vi "y1y2 (子VI)-2.vi"(11 "Image Pixels (U8)输入":u8[][](array[numeric])) -> (0 "输出数组 2":cluster{i32, i32}[](array[cluster]), 2 "输出数组":cluster{i32, i32}[](array[cluster]))   [LabVIEW 2014]
panel:
  out "元素索引 2":i32
  out "元素索引":i32
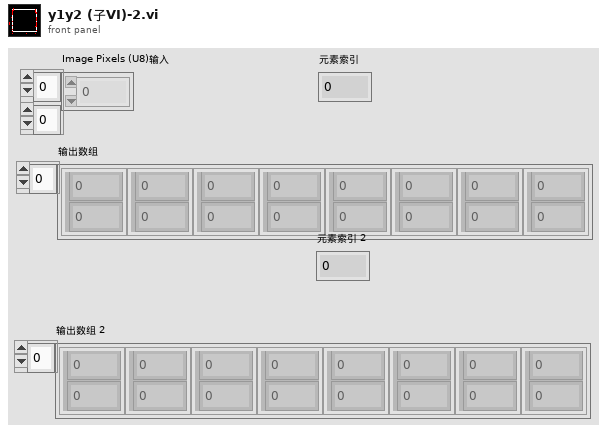
[diagram p1: front panel]
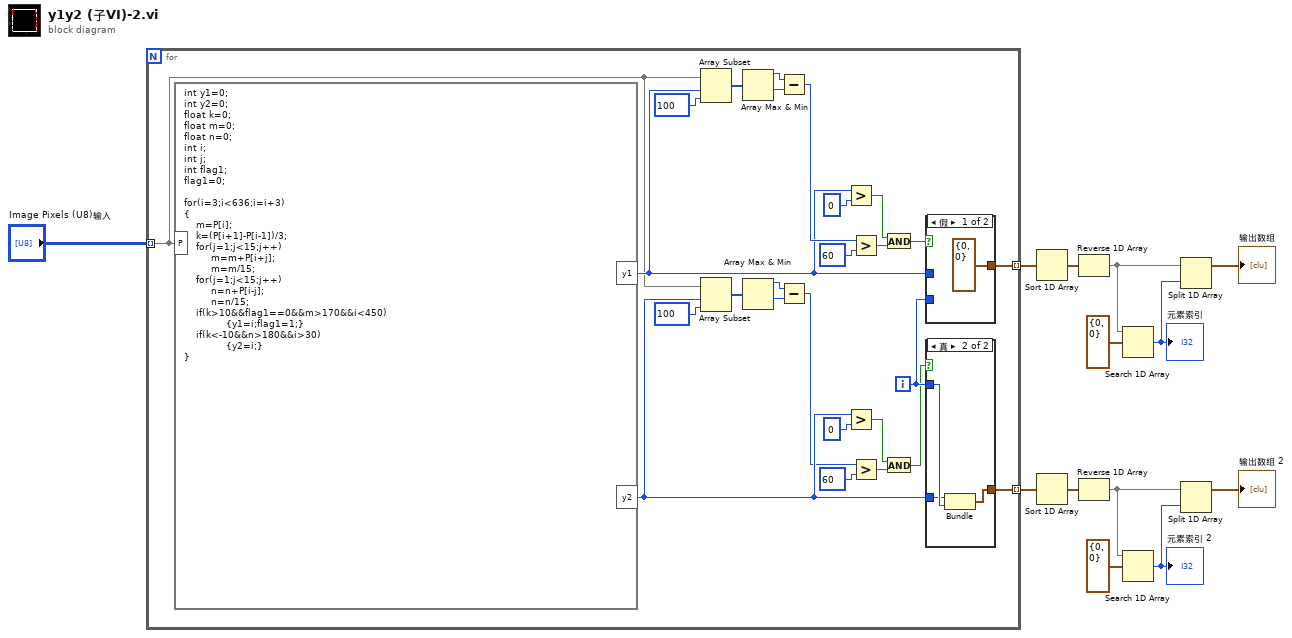
[diagram p0: block diagram]
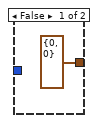
[diagram p2: hidden frame]
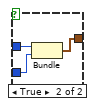
[diagram p3: hidden frame]
diagram:
  n1 = for {
    tunnel: "Image Pixels (U8)输入" -> [w16] mode=indexing
    tunnel: [w39] -> w1 mode=indexing
    tunnel: [w38] -> w7 mode=indexing
    i -> [w37]
    n2 = formula code="int y1=0;\nint y2=0;\nfloat k=0;\nfloat m=0;\nfloat n=0;\nint i;\nint j;\nint flag1;\nflag1=0;\n\nfor(i=3;i<636;i=i+3)\n{\n    m=P[i];\n    k=(P[i+1]-P[i-1])/3;\n    for(j=1;j<15;j++)\n         m=m+P[i+j];\n         m=m/15;\n    for(j=1;j<15;j++)\n         n=n+P[i-j];\n         n=n/15;\n    if(k>10&&flag1==0&&m>170&&i<450)\n              {y1=i;flag1=1;}\n    if(k<-10&&n>180&&i>30)\n              {y2=i;}\n}"("P"=w16) -> ("y1"=w17:i32, "y2"=w28:i32)
    n3 = Array Subset(array=w16, index=w17, length=100 ("长度")) -> (w19:u8[])
    n4 = Array Subset(array=w16, index=w28, length=100 ("长度")) -> (w33:u8[])
    n5 = Array Max & Min(array=w19) -> (max value=w20:u8, min value=w21:u8)  [unwired: 2 out]
    n6 = Array Max & Min(array=w33) -> (max value=w32:u8, min value=w31:u8)  [unwired: 2 out]
    n7 = Subtract(x=w20, y=w21) -> (x-y=w22:u8)
    n8 = Subtract(x=w32, y=w31) -> (x-y=w27:u8)
    n9 = Greater?(x=w17, y=0) -> (0:w15:bool)
    n10 = Greater?(x=w28, y=0) -> (0:w30:bool)
    n11 = Greater?(x=w22, y=u8 60) -> (0:w24:bool)
    n12 = Greater?(x=w27, y=u8 60) -> (0:w25:bool)
    n13 = And(x=w15, y=w24) -> (x .and. y?=w14:bool)
    n14 = And(x=w30, y=w25) -> (x .and. y?=w29:bool)
    n15 = case shown="假" w14 {
      tunnel: [cluster{i32, i32} {0, 0} w47] -> w38
      tunnel: w37 -> [_ w46]
      tunnel: w17 -> [_ w45]
      frame False {
      }
      frame True {
        n16 = Bundle(w45, w46) -> (w47:cluster{i32, i32})  [unwired: 1 in]
      }
    }
    n17 = case shown="真" w29 {
      tunnel: [cluster{i32, i32} {0, 0} w43] -> w39
      tunnel: w37 -> [_ w42]
      tunnel: w28 -> [_ w41]
      frame False {
      }
      frame True {
        n18 = Bundle(w41, w42) -> (w43:cluster{i32, i32})  [unwired: 1 in]
      }
    }
  }
  n19 = Sort 1D Array(array=w7) -> (sorted array=w12:cluster{i32, i32}[])
  n20 = Sort 1D Array(array=w1) -> (sorted array=w2:cluster{i32, i32}[])
  n21 = Reverse 1D Array(array=w12) -> (reversed array=w9:cluster{i32, i32}[])
  n22 = Reverse 1D Array(array=w2) -> (reversed array=w5:cluster{i32, i32}[])
  n23 = Search 1D Array(1D array=w9, element=cluster{i32, i32} {0, 0} ("元素")) -> (index of element=w10:i32)  [unwired: 1 in]
  "元素索引" <- w10
  n24 = Search 1D Array(1D array=w5, element=cluster{i32, i32} {0, 0} ("元素")) -> (index of element=w4:i32)  [unwired: 1 in]
  "元素索引 2" <- w4
  n25 = Split 1D Array(array=w9, index=w10) -> (first subarray=→"输出数组":cluster{i32, i32}[])  [unwired: 1 out]
  n26 = Split 1D Array(array=w5, index=w4) -> (first subarray=→"输出数组 2":cluster{i32, i32}[])  [unwired: 1 out]
